vi "VARIENT_TO_DATA.vi"(2 "data":variant[][](array[variant]), 3 "error in (no error)":errorcluster) -> (7 "Table":string[][](array[string]), 10 "error out":errorcluster)   [LabVIEW 2017]
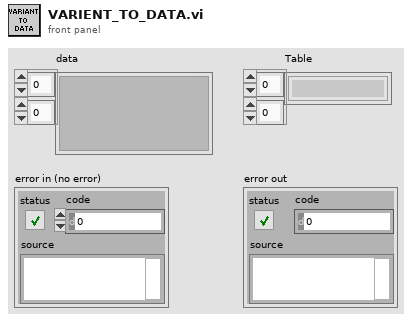
[diagram p1: front panel]
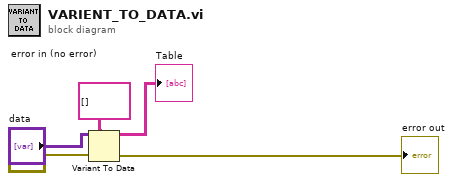
[diagram p0: block diagram]
diagram:
  n1 = Variant To Data(error in="error in (no error)", type=string[][] [] ("Table"), Variant="data") -> (data=→"Table":string[][], error out=→"error out":errorcluster)
